vi "TriggerTheCamera.vi"(0 "seconds to wait":u32=1200, 11 "error out 2":errorcluster) -> (15 "error out":errorcluster)   [LabVIEW 2011]
uses:
  <vilib>/DAQmx/write.llb/DAQmx Write (Digital Bool 1Line 1Point).vi
  <vilib>/DAQmx/create/channels.llb/DAQmx Create Channel (DO-Digital Output).vi
  <vilib>/DAQmx/miscellaneous.llb/DAQmx Fill In Error Info.vi
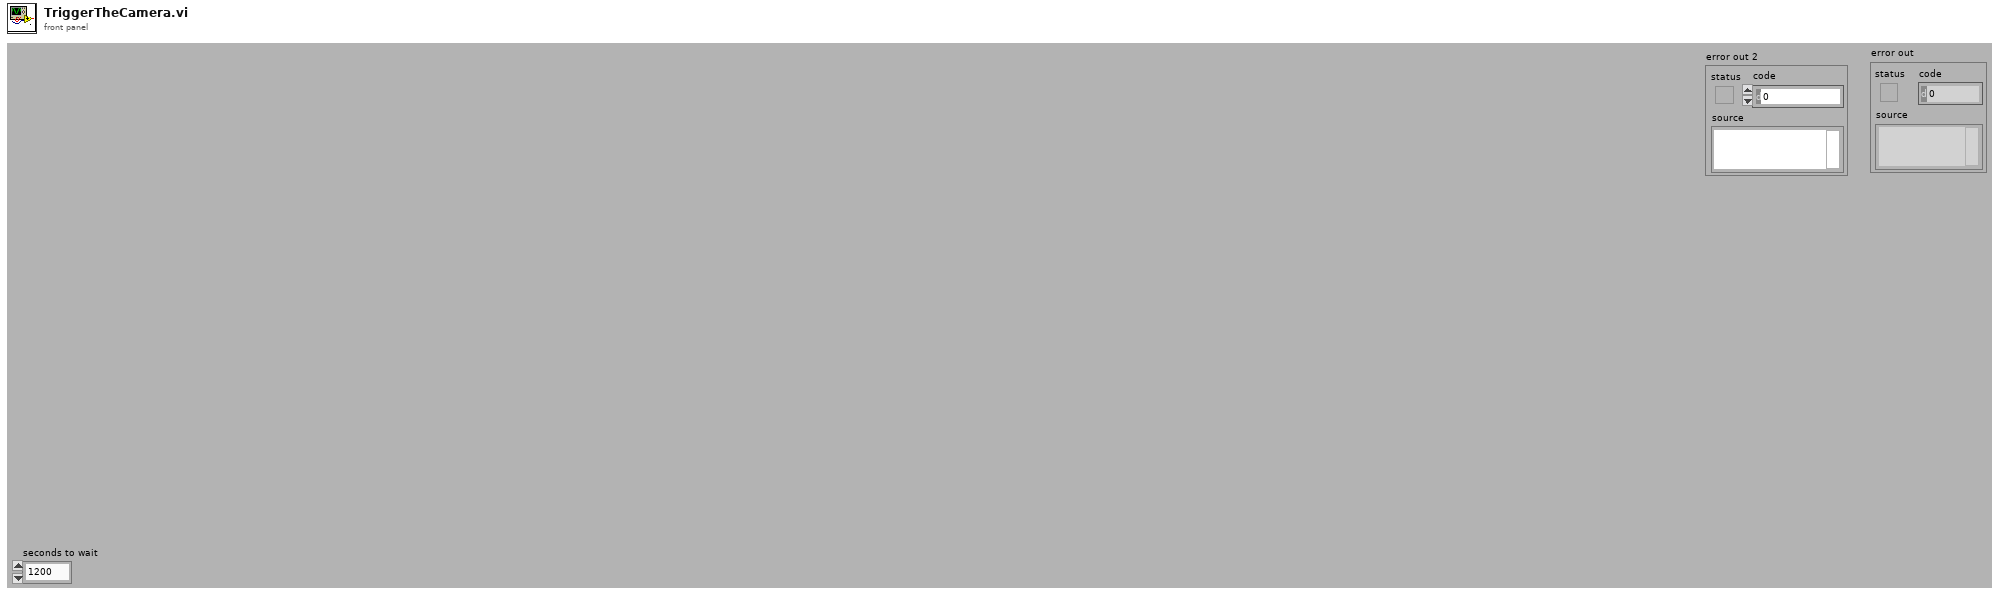
[diagram p1: front panel]
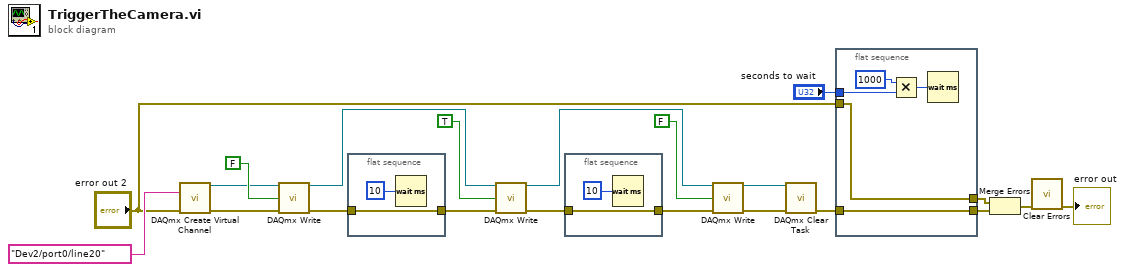
[diagram p0: block diagram]
diagram:
  n1 = call-poly <vilib>:"DAQmx Create Virtual Channel.vi"("lines"=tag "Dev2/port0/line20", "error in"="error out 2") -> ("task out"=w11:refnum<k21>, "error out"=w14:errorcluster)  [unwired: 12 in]
  n2 = call-poly <vilib>:"DAQmx Write.vi"("task/channels in"=w11, "data"=FALSE, "error in"=w14) -> ("task out"=w10:refnum<k21>, "error out"=w6:errorcluster)  [unwired: 10 in, 1 out]
  n3 = flat-sequence {
    tunnel: [w23] -> w7
    tunnel: w6 -> [w23]
    frame #0 {
      n4 = Wait (ms)(milliseconds to wait=u32 10) -> ()  [unwired: 1 out]
    }
  }
  n5 = call-poly <vilib>:"DAQmx Write.vi"("task/channels in"=w10, "data"=TRUE, "error in"=w7) -> ("task out"=w9:refnum<k21>, "error out"=w4:errorcluster)  [unwired: 10 in, 1 out]
  n6 = flat-sequence {
    tunnel: [w25] -> w5
    tunnel: w4 -> [w25]
    frame #0 {
      n7 = Wait (ms)(milliseconds to wait=u32 10) -> ()  [unwired: 1 out]
    }
  }
  n8 = call-poly <vilib>:"DAQmx Write.vi"("task/channels in"=w9, "data"=FALSE, "error in"=w5) -> ("task out"=w8:refnum<k21>, "error out"=w12:errorcluster)  [unwired: 10 in, 1 out]
  n9 = call <vilib>:"DAQmx Clear Task.vi"("task in"=w8, "error in"=w12) -> ("error out"=w1:errorcluster)  [unwired: 13 in]
  n10 = flat-sequence {
    tunnel: "error out 2" -> [w30]
    tunnel: [w30] -> w19
    tunnel: "seconds to wait" -> [w29]
    tunnel: [w26] -> w2
    tunnel: w1 -> [w26]
    frame #0 {
      n11 = Multiply(x=u32 1000, y=w29) -> (x*y=w27:u32)
      n12 = Wait (ms)(milliseconds to wait=w27) -> ()  [unwired: 1 out]
    }
  }
  n13 = Merge Errors(w19, w2) -> (w18:errorcluster)
  n14 = call <vilib>:"Clear Errors.vi"("error in (no error)"=w18) -> ("error out"=→"error out":errorcluster)  [unwired: 6 in]
